vi "Write Include Title.vi"(8 "error in (no error)":errorcluster, 10 "Include Title?":bool, 11 "PieChart in":refnum<class "PieChart.lvclass">) -> (0 "error out":errorcluster, 3 "PieChart out":refnum<class "PieChart.lvclass">)   [LabVIEW 2020, in "PieChart.lvclass"]
uses:
  PieChart.lvclass
  PieChart.lvclass/PieChart.ctl
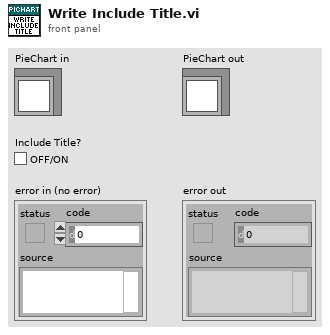
[diagram p1: front panel]
types:
  T1 = typedef "PieChart.lvclass/State Data.ctl" = cluster{"Title":string, "Values[]":dbl[], "Labels[]":string[], "Colors[]":u32[], "Include Legend?":bool, "Include Title?":bool, "Title Font":T2, "Legend Font":T2, "Selection":i32, "Slice Positions":T3}
  T2 = typedef "LVFontTypeDef.ctl" = cluster{"Font Name":string, "Size":u16, "Bold":bool, "Italic":bool, "Underline":bool, "Strikeout":bool, "Color":u32}
  T3 = typedef "PieChart.lvclass/Pie info for Click.ctl" = cluster{"Slice Positions":cluster{"Start":i16, "End":i16}[], "Center Position":T4, "Radius":i16}
  T4 = typedef "LVBoundsTypeDef.ctl" = cluster{"Width":u32, "Height":u32}
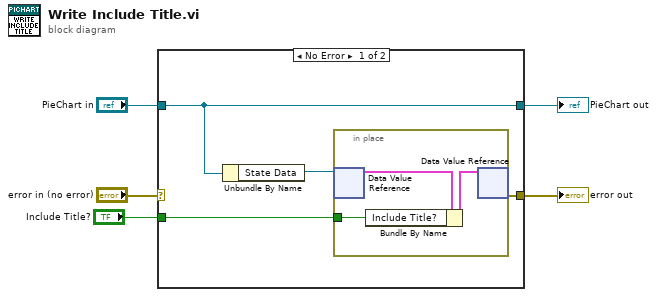
[diagram p0: block diagram]
diagram:
  n1 = case shown="No Error" "error in (no error)" {
    selector: "error in (no error)" -> [_ w14]
    tunnel: [w6 w14] -> w4
    tunnel: [w7 w13] -> w2
    tunnel: "PieChart in" -> [w7 w13]
    tunnel: "Include Title?" -> [w9 _]
    frame No Error {
      n2 = Unbundle By Name(w7) -> ("State Data"=w8:refnum<data-value>)
      n3 = in-place {
        in-place-border: w9 -> [w10]
        n4 = in-place-dvr #1(w8) -> (w12:T1)  [unwired: 1 out]
        n5 = Bundle By Name(cluster=w12, "Include Title?"=w10) -> (w11:T1)
        n6 = in-place-dvr #1(w11) -> (w6:errorcluster)  [unwired: 1 out]
      }
    }
    frame Error {
    }
  }
  "error out" <- w4
  "PieChart out" <- w2
